vi "dospi_1394_grises.vi"() -> (0 "dt (ms) 2":u16=5, 1 "Canal 2":string="X", 2 "InterfaceName":string="cam0", 3 "Puerto 2":refnum<visa-resource-name>="COM2", 4 "Selección Rectángulo (px) 2":T1={"Left"=80, "Top"=180, "Right"=730, "Bottom"=830}, 5 "V 2Pi\nActual":sgl=3.4309938 format="%#.1g")   [LabVIEW 2020]
uses:
  <vilib>/Instr/_visa.llb/VISA Find Search Mode.ctl
  <vilib>/Instr/_visa.llb/VISA Configure Serial Port (Instr).vi
  <vilib>/vision/NI_Vision_Development_Module.lvlib
  <vilib>/gmath/NI_Gmath.lvlib
  <vilib>/vision/driver/NI_Vision_Acquisition_Software.lvlib
  <vilib>/Analysis/NI_AAL_SigProc.lvlib
panel:
  in  "Sust":bool=TRUE
  in  "Sustracción 2":bool
  in  "V 2Pi\nApriori":sgl=4.0 min=0.1 max=15 step=0.1 format="%.1f"
  in  "Puerto":refnum<visa-resource-name>="COM2"
  in  "Selección Rectángulo (px)":T1={"Left"=80, "Top"=180, "Right"=730, "Bottom"=830}
  in  "dV (V)":sgl=0.4 min=0.1 max=5 step=0.1 format="%.1f"
  in  "dt (ms)":u16=5
  in  "Rango (V)":u8=7 max=100 step=1
  in  "Canal":string="X"
  out "valor enviado":string="17.2"
  in  "Sustracción":bool
  out "Captura":T2(plugin-control)
  in  "error in (no error)":errorcluster
  out "tiempo total":u32=1016
  out "Ciclos 2Pi":cluster{"xi used":dbl[], "yi":dbl[]}[](graph)=[{"xi used"=[0.0, 0.4000000059604645, 0.800000011920929, 1.2000000476837158, 1.600000023841858, 2.0, 2.4000000953674316, 2.799999952316284, 3.200000047683716, 3.6000001430511475, 4.0, 4.400000095367432, 4.800000190734863, 5.200000286102295, 5.599999904632568, 6.0, 6.400000095367432, 6.800000190734863, 7.200000286102295], "yi"=[1.6194082498550415, 2.081223726272583, 3.9639101028442383, 5.417988300323486, 5.994996547698975, 5.763517379760742, 4.927460193634033, 3.268064022064209, 1.9228070974349976, 2.006049633026123, 3.322584629058838, 5.178757190704346, 5.874281883239746, 5.9817633628845215, 5.3586106300354, 3.7743194103240967, 2.4187028408050537, 2.3153183460235596, 3.7917206287384033]}, {"xi used"=[0.0, 0.10000000149011612, 0.20000000298023224, 0.30000000447034836, 0.4000000059604645, 0.5000000074505806, 0.6000000089406967, 0.7000000104308128, 0.800000011920929, 0.9000000208616257, 1.0000000298023224, 1.100000038743019, 1.2000000476837158, 1.3000000417232513, 1.4000000357627869, 1.5000000298023224, 1.600000023841858, 1.7000000178813934, 1.800000011920929, 1.9000000059604645, 2.0, 2.100000023841858, 2.200000047683716, 2.3000000715255737, 2.4000000953674316, 2.5000000596046448, 2.600000023841858, 2.699999988079071, 2.799999952316284, 2.899999976158142, 3.0, 3.100000023841858, 3.200000047683716, 3.3000000715255737, 3.4000000953674316, 3.5000001192092896, 3.6000001430511475, 3.7000001072883606, 3.8000000715255737, 3.900000035762787, 4.0, 4.100000023841858, 4.200000047683716, 4.300000071525574, 4.400000095367432, 4.5000001192092896, 4.6000001430511475, 4.700000166893005, 4.800000190734863, 4.900000214576721, 5.000000238418579, 5.100000262260437, 5.200000286102295, 5.300000190734863, 5.400000095367432, 5.5, 5.599999904632568, 5.699999928474426, 5.799999952316284, 5.899999976158142, 6.0, 6.100000023841858, 6.200000047683716, 6.300000071525574, 6.400000095367432, 6.5000001192092896, 6.6000001430511475, 6.700000166893005, 6.800000190734863, 6.900000214576721, 7.000000238418579, 7.100000262260437, 7.200000286102295], "yi"=[1.6194082498550415, 1.6415202646400873, 1.700969021152869, 1.835091261121122, 2.081223726272583, 2.4615675244221595, 2.9377812277334487, 3.4563877744572187, 3.9639101028442383, 4.416314498578613, 4.807340439884618, 5.1401707620402455, 5.417988300323486, 5.643229129866736, 5.815342479071086, 5.9330308007455095, 5.994996547698975, 6.0015645873541725, 5.959549445588673, 5.8773880628937665, 5.763517379760742, 5.622745854472534, 5.4453682711596425, 5.218050945615625, 4.927460193634033, 4.566549653810085, 4.153420905030226, 3.7124627576598135, 3.268064022064209, 2.8442846434260165, 2.4638706226251452, 2.1492390703865025, 1.9228070974349976, 1.8016579460584699, 1.7815393847964844, 1.8528653137515367, 2.006049633026123, 2.2327082258196134, 2.529265762805696, 2.8933489839101707, 3.322584629058838, 3.807336769827714, 4.308917005977046, 4.78137419407865, 5.178757190704346, 5.467236063197128, 5.661465721984701, 5.788222288265946, 5.874281883239746, 5.940712665430707, 5.985750942666336, 6.001925060099863, 5.9817633628845215, 5.9173299887642, 5.798831744986865, 5.616011126946077, 5.3586106300354, 5.0225638976458455, 4.628571701943094, 4.203526165358669, 3.7743194103240967, 3.3657338746848104, 2.994113257941885, 2.673691575010305, 2.4187028408050537, 2.2430304554985607, 2.1591553602930404, 2.1792078816481535, 2.3153183460235596, 2.5722541809073114, 2.925331217901028, 3.3425023896347215, 3.7917206287384033]}, {"xi used"=[1.6635191881348852, 5.094512955533968], "yi"=[6.004797437208987, 6.001979760925586]}]
  out "error out":errorcluster
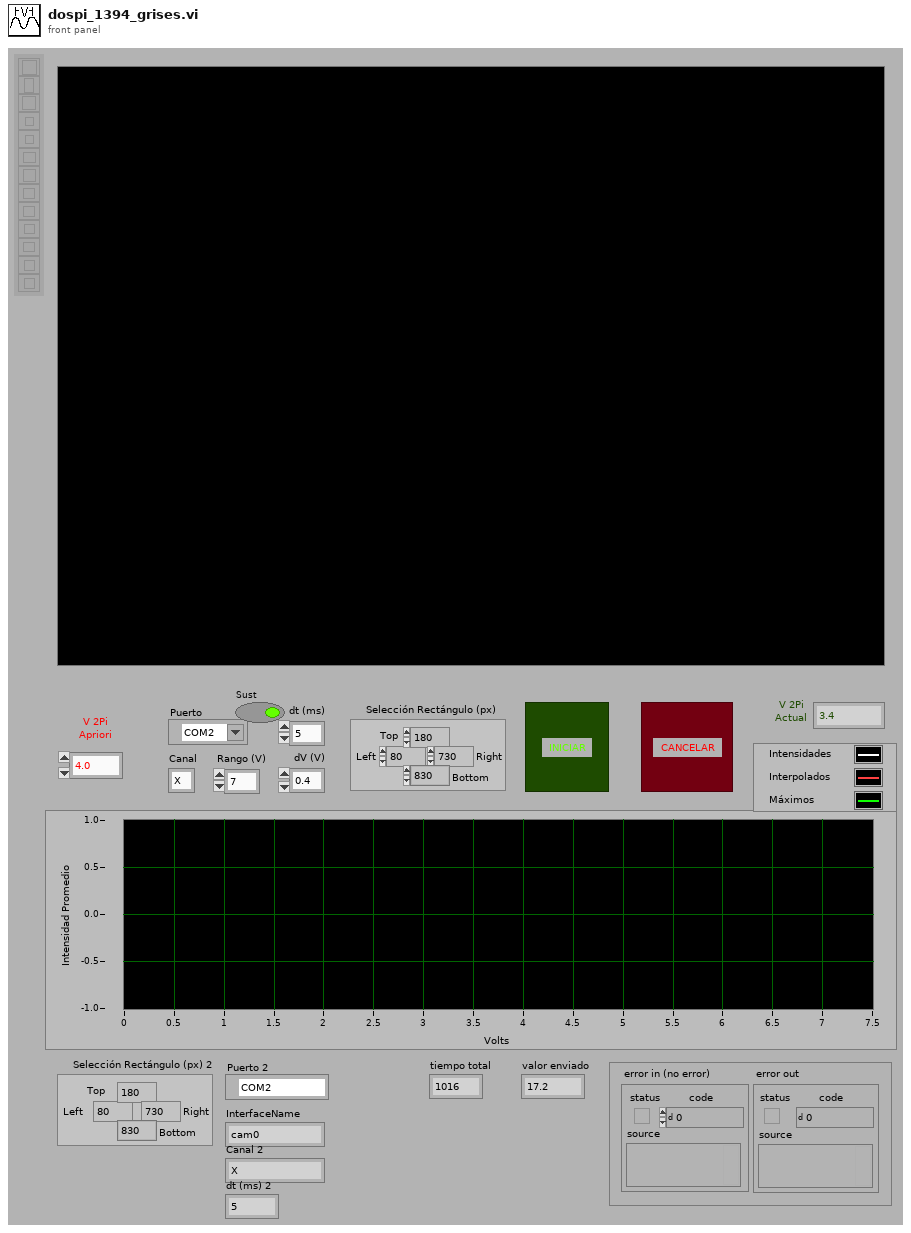
[diagram p1: front panel]
types:
  T1 = cluster{"Left":i32, "Top":i32, "Right":i32, "Bottom":i32}
  T2 = typedef "IMAQ Image.ctl" = refnum<image>
  T3 = typedef "VISA Find Search Mode.ctl" = u32
  T4 = cluster{"Type":u32, "Version":u32, "Flags":u32, "SerialNumberHigh":u32, "SerialNumberLow":u32, "BusType":u32, "InterfaceName":string, "VendorName":string, "ModelName":string, "CameraFileName":string, "CameraAttributeURL":string}[]
  T5 = cluster{"Type":u32, "Version":u32, "Flags":u32, "SerialNumberHigh":u32, "SerialNumberLow":u32, "BusType":u32, "InterfaceName":string, "VendorName":string, "ModelName":string, "CameraFileName":string, "CameraAttributeURL":string}
  T6 = typedef "IMAQdx.ctl" = refnum<k21>
  T7 = cluster{"Mean Value":sgl, "Standard Variation":sgl, "Minimal Value":sgl, "Maximal Value":sgl, "Area (calibrated)":sgl, "Area (pixels)":i32, "%":sgl}
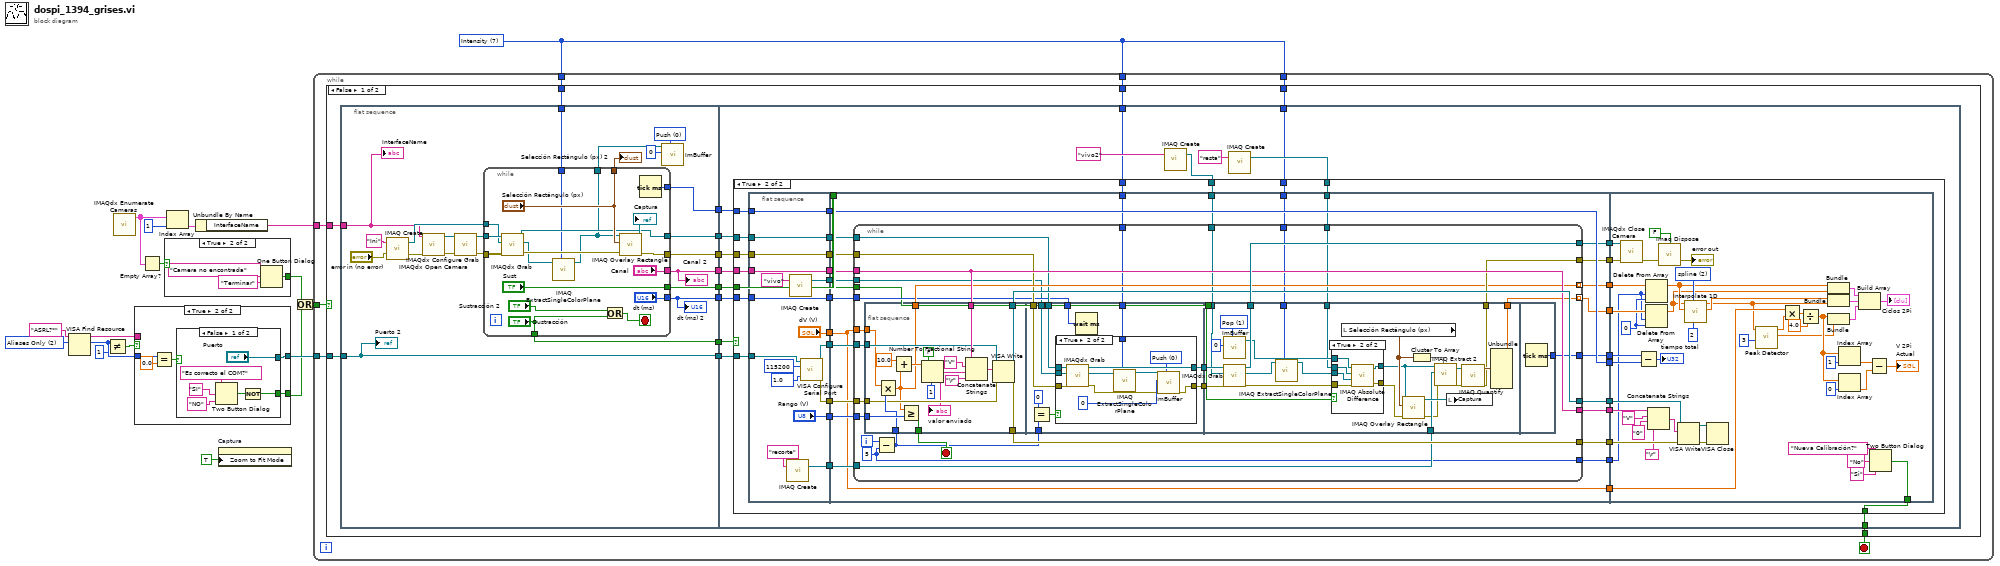
[diagram p0: block diagram]
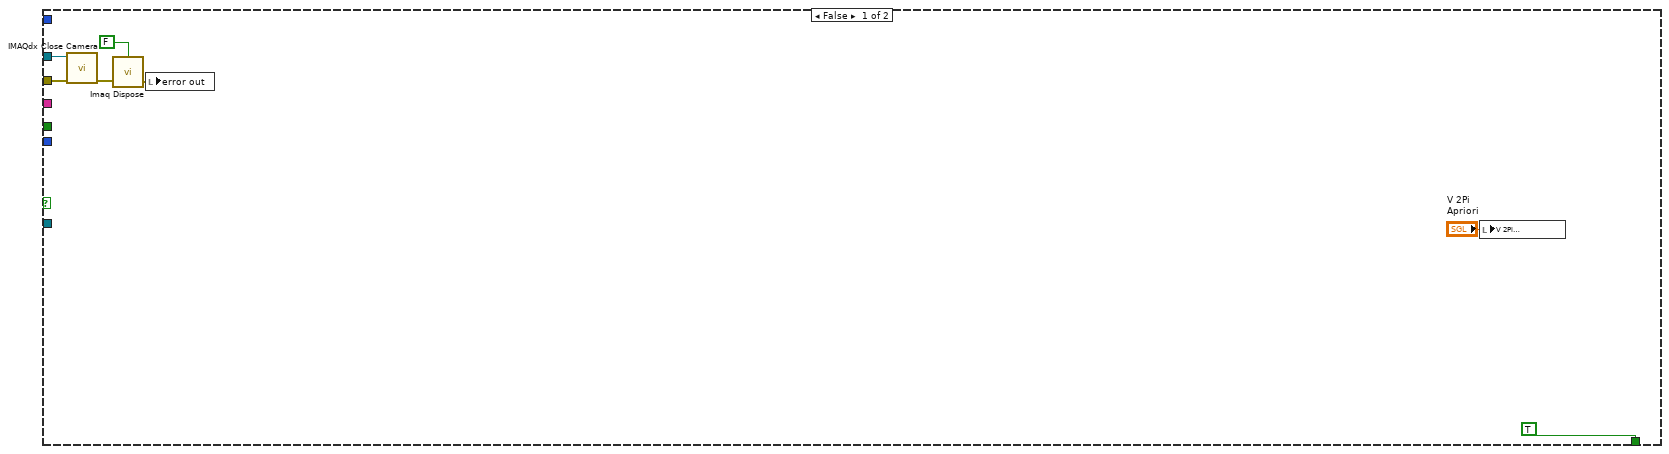
[diagram p2: hidden frame]
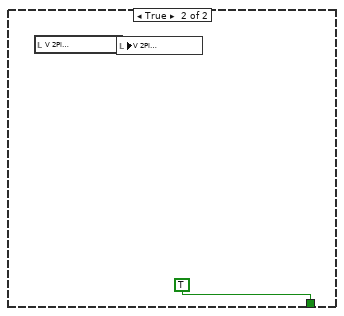
[diagram p5: hidden frame]
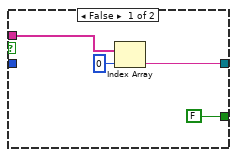
[diagram p6: hidden frame]
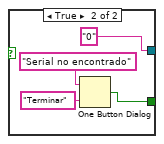
[diagram p7: hidden frame]
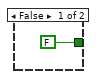
[diagram p8: hidden frame]
diagram:
  w1 = 7 items=["Red", "Green", "Blue", "Hue", "Saturation", "Luminance", "Value", "Intensity"] ("Color Plane")
  w12 = T3 2 items=["Canonical Names Only"=0, "Aliases Only"=2, "Include Matching Aliases"=3, "Include All Aliases"=4] ("Search Mode")
  n1 = VISA Find Resource(10:w12, 11:"ASRL?*" ("expression (\"?*\")")) -> (2:w17:u32, 3:w16:string[])  [unwired: 1 in, 1 out]
  n2 = Not Equal?(x=w17, y=u32 1) -> (x != y?=w15:bool)
  n3 = call <vilib>:"IMAQdx Enumerate Cameras.vi"() -> ("Camera Information Array"=w10:T4)  [unwired: 10 in, 1 out]
  n4 = case shown="True" w15 {
    tunnel: w16 -> [w21 _]
    tunnel: [w19 w26] -> w6
    tunnel: w17 -> [_ w24]
    tunnel: [FALSE ("true") w22] -> w4
    frame False {
      n5 = Index Array(array=w21, index=0) -> (element=w19:string)
    }
    frame True {
      n6 = Equal?(x=w24, y=0.0) -> (x = y?=w23:bool)
      n7 = case shown="False" w23 {
        tunnel: ["Puerto" "0" ("button name (\"OK\")")] -> w26
        tunnel: [w27 w33] -> w22
        frame False {
          n8 = Two Button Dialog(message="Es correcto el COM?" ("error source (\" \")"), 1:"NO" ("F button name (\"Cancel\")"), 2:"SI" ("T button name (\"OK\")")) -> (T button?=w28:bool)
          n9 = Not(x=w28) -> (.not. x?=w27:bool)
        }
        frame True {
          n10 = One Button Dialog(message="Serial no encontrado" ("error source (\" \")"), button name ("OK")="Terminar") -> (true=w33:bool)
        }
      }
    }
  }
  n11 = Empty Array?(array=w10) -> (empty?=w11:bool)
  n12 = case shown="True" w11 {
    tunnel: [FALSE ("true") w38] -> w5
    frame False {
    }
    frame True {
      n13 = One Button Dialog(message="Camera no encontrada" ("error source (\" \")"), button name ("OK")="Terminar") -> (true=w38:bool)
    }
  }
  n14 = Index Array(array=w10, index=1) -> (element=w9:T5)
  n15 = Unbundle By Name(w9) -> ("InterfaceName"=w7:string)
  n16 = property on="Captura" class="ImageControl"("Zoom to Fit Mode"=TRUE) -> ()  [unwired: 2 in, 2 out]
  n17 = Or(x=w5, y=w4) -> (x .or. y?=w3:bool)
  n18 = while {
    tunnel: w7 -> [w47]
    tunnel: w6 -> [w46]
    tunnel: w3 -> [w45]
    tunnel: w1 -> [w43]
    tunnel: w1 -> [w42]
    tunnel: w1 -> [w41]
    stop <- w44 stop-if-true
    n19 = case shown="False" w45 {
      tunnel: w47 -> [w61 _]
      tunnel: w46 -> [w60 _]
      tunnel: [w52 TRUE ("T button?")] -> w44
      tunnel: w43 -> [w50 _]
      tunnel: w42 -> [w49 _]
      tunnel: w41 -> [w48 _]
      frame False {
        n20 = flat-sequence {
          tunnel: w61 -> [w75]
          tunnel: w60 -> [w68]
          tunnel: [w68] -> w59
          tunnel: [w74] -> w58
          tunnel: [w73] -> w57
          tunnel: [w72] -> w56
          tunnel: [w71] -> w55
          tunnel: [w70] -> w54
          tunnel: [w69] -> w53
          tunnel: [w63] -> w51
          tunnel: w50 -> [w62]
          tunnel: w59 -> [w116]
          tunnel: w58 -> [w115]
          tunnel: w57 -> [w114]
          tunnel: w56 -> [w113]
          tunnel: w55 -> [w112]
          tunnel: w54 -> [w111]
          tunnel: w53 -> [w110]
          tunnel: [w109] -> w52
          tunnel: w51 -> [w104]
          tunnel: w49 -> [w103]
          tunnel: w48 -> [w102]
          frame #0 {
            w65 = u16 0 items=["Push", "Pop", "Reset"] ("Function")
            n21 = call "IMAQ Create"("Image Name"="Ini", "error in (no error)"="error in (no error)") -> ("New Image"=w79:T2, "error out"=w76:errorcluster)  [unwired: 3 in]
            n22 = call <vilib>:"IMAQdx Open Camera.vi"("error in"=w76, "Session In"=w75) -> ("error out"=w77:errorcluster, "Session Out"=w78:T6)  [unwired: 8 in]
            n23 = call <vilib>:"IMAQdx Configure Grab.vi"("error in"=w77, "Session In"=w78) -> ("error out"=w80:errorcluster, "Session Out"=w81:T6)  [unwired: 8 in]
            n24 = while {
              tunnel: w80 -> [w100]
              tunnel: [w89] -> w73
              tunnel: w81 -> [w101]
              tunnel: w79 -> [w99]
              tunnel: [w98] -> w74
              tunnel: [w91] -> w72
              tunnel: ["Sustracción"] -> w71
              tunnel: ["Canal"] -> w70
              tunnel: ["dt (ms)"] -> w69
              tunnel: [w85] -> w66
              tunnel: ["Selección Rectángulo (px)"] -> w67
              tunnel: ["Sust"] -> w63
              tunnel: w62 -> [w84]
              stop <- w97 stop-if-true
              n25 = call <vilib>:"IMAQdx Grab.vi"("error in"=w100, "Image In"=w99, "Session In"=w101) -> ("error out"=w87:errorcluster, "Image Out"=w86:T2, "Session Out"=w89:T6)  [unwired: 5 in, 1 out]
              n26 = call "IMAQ ExtractSingleColorPlane"("Color Plane"=w84, "Image Src"=w86) -> ("Image Dst Out"=w85:T2)  [unwired: 8 in, 1 out]
              n27 = Or(x="Sustracción 2", y="Sustracción") -> (x .or. y?=w97:bool)
              n28 = call "IMAQ Overlay Rectangle"("error in (no error)"=w87, "Rectangle"="Selección Rectángulo (px)", "Image"=w85) -> ("error out"=w91:errorcluster, "Image Out"=→"Captura":T2)  [unwired: 7 in]
              n29 = Tick Count (ms)() -> (millisecond timer value=w98:u32)
            }
            "Canal 2" <- w70
            "dt (ms) 2" <- w69
            "Selección Rectángulo (px) 2" <- w67
            n30 = call "ImBuffer.vi"("Function"=w65, "Buffer #"=0, "Image In"=w66) -> ()  [unwired: 6 in, 3 out]
            "Puerto 2" <- w68
            "InterfaceName" <- w75
          }
          frame #1 {
            n31 = call "IMAQ Create"("Image Name"="vivo2") -> ("New Image"=w105:T2)  [unwired: 4 in, 1 out]
            n32 = call "IMAQ Create"("Image Name"="resta") -> ("New Image"=w107:T2)  [unwired: 4 in, 1 out]
            n33 = case shown="True" w112 {
              tunnel: w116 -> [_ w136]
              tunnel: w115 -> [_ w135]
              tunnel: w114 -> [w123 w134]
              tunnel: w113 -> [w122 w133]
              tunnel: w111 -> [_ w132]
              tunnel: w110 -> [_ w130]
              tunnel: [TRUE ("T button?") w129] -> w109
              tunnel: w107 -> [_ w128]
              tunnel: w105 -> [_ w127]
              tunnel: w104 -> [_ w126]
              tunnel: w103 -> [_ w125]
              tunnel: w102 -> [_ w124]
              frame False {
                n34 = call <vilib>:"IMAQdx Close Camera.vi"("error in"=w122, "Session In"=w123) -> ("error out"=w119:errorcluster)  [unwired: 9 in]
                n35 = call "Imaq Dispose"("All Images? (No)"=FALSE, "error in (no error)"=w119) -> ("error out"=w117:errorcluster)  [unwired: 4 in]
                n36 = local write "error out"(w117) -> ()
                n37 = local write "V 2Pi\nActual"("V 2Pi\nApriori") -> ()
              }
              frame True {
                n38 = flat-sequence {
                  tunnel: ["Rango (V)"] -> w157
                  tunnel: [w158] -> w156
                  tunnel: [w163] -> w155
                  tunnel: [w162] -> w154
                  tunnel: [w164] -> w153
                  tunnel: [w166] -> w152
                  tunnel: [w161] -> w151
                  tunnel: [w169] -> w150
                  tunnel: [w168] -> w149
                  tunnel: ["dV (V)"] -> w148
                  tunnel: w136 -> [w165]
                  tunnel: w135 -> [w164]
                  tunnel: w134 -> [w163]
                  tunnel: w133 -> [w162]
                  tunnel: w132 -> [w161]
                  tunnel: [w160] -> w131
                  tunnel: w130 -> [w160]
                  tunnel: w157 -> [w181]
                  tunnel: w156 -> [w197]
                  tunnel: w155 -> [w198]
                  tunnel: w154 -> [w196]
                  tunnel: w153 -> [w195]
                  tunnel: [w195] -> w147
                  tunnel: [w194] -> w146
                  tunnel: [w193] -> w145
                  tunnel: [w192] -> w144
                  tunnel: [w191] -> w143
                  tunnel: [w190] -> w142
                  tunnel: [w189] -> w141
                  tunnel: [w188] -> w140
                  tunnel: [w187] -> w139
                  tunnel: w152 -> [w186]
                  tunnel: w151 -> [w185]
                  tunnel: w150 -> [w183]
                  tunnel: w149 -> [w184]
                  tunnel: [w182] -> w138
                  tunnel: w148 -> [w180]
                  tunnel: [w180] -> w137
                  tunnel: w131 -> [w179]
                  tunnel: w128 -> [w178]
                  tunnel: w127 -> [w177]
                  tunnel: w126 -> [w176]
                  tunnel: w125 -> [w175]
                  tunnel: w124 -> [w174]
                  tunnel: w147 -> [w343]
                  tunnel: w146 -> [w347]
                  tunnel: w145 -> [w346]
                  tunnel: w144 -> [w345]
                  tunnel: w143 -> [w344]
                  tunnel: w142 -> [w333]
                  tunnel: w141 -> [w341]
                  tunnel: w140 -> [w342]
                  tunnel: w139 -> [w335]
                  tunnel: w138 -> [w331]
                  tunnel: w137 -> [w328]
                  tunnel: [w313] -> w129
                  frame #0 {
                    w171 = u16 10 items=["1.0"=10, "1.5"=15, "2.0"=20] ("stop bits (10: 1 bit)")
                    n39 = call "IMAQ Create"("Image Name"="recorte") -> ("New Image"=w166:T2)  [unwired: 4 in, 1 out]
                    n40 = call "IMAQ Create"("Image Name"="vivo") -> ("New Image"=w158:T2)  [unwired: 4 in, 1 out]
                    n41 = call-poly "VISA Configure Serial Port"("VISA resource name"=w165, "baud rate (9600)"=u32 115200, "stop bits (10: 1 bit)"=w171) -> ("VISA resource name out"=w168:refnum<visa-resource-name>, "error out"=w169:errorcluster)  [unwired: 11 in]
                  }
                  frame #1 {
                    n42 = while {
                      tunnel: [w217] -> w190 mode=indexing
                      tunnel: [w221] -> w194
                      tunnel: w185 -> [w221]
                      tunnel: [w222] -> w193
                      tunnel: w184 -> [w223]
                      tunnel: w183 -> [w224]
                      tunnel: w181 -> [w225]
                      tunnel: [w226] -> w192
                      tunnel: w196 -> [w207]
                      tunnel: w197 -> [w203]
                      tunnel: w198 -> [w208]
                      tunnel: [w220] -> w191
                      tunnel: [w214] -> w189
                      tunnel: [w219] -> w188
                      tunnel: [w218] -> w187 mode=indexing
                      tunnel: w186 -> [w216]
                      tunnel: [w212] -> w182
                      tunnel: w180 -> [w211]
                      tunnel: w179 -> [w204]
                      tunnel: w178 -> [w210]
                      tunnel: w177 -> [w202]
                      tunnel: w176 -> [w201]
                      tunnel: w175 -> [w200]
                      tunnel: w174 -> [w199]
                      i -> [w213]
                      stop <- w215 stop-if-true
                      w212 = 5 ("x")
                      n43 = flat-sequence {
                        tunnel: w223 -> [w231]
                        tunnel: w224 -> [w234]
                        tunnel: [w242] -> w215
                        tunnel: w209 -> [w239]
                        tunnel: w225 -> [w241]
                        tunnel: w221 -> [w233]
                        tunnel: [w227] -> w218
                        tunnel: [w230] -> w222
                        tunnel: [w229] -> w219
                        tunnel: w211 -> [w228]
                        tunnel: w204 -> [w254]
                        tunnel: w209 -> [w252]
                        tunnel: w208 -> [w250]
                        tunnel: w207 -> [w249]
                        tunnel: [w248] -> w206
                        tunnel: [w247] -> w205
                        tunnel: w203 -> [w246]
                        tunnel: w200 -> [w245]
                        tunnel: [w288] -> w226
                        tunnel: [w287] -> w220
                        tunnel: [w286] -> w217
                        tunnel: w216 -> [w285]
                        tunnel: w210 -> [w275]
                        tunnel: w206 -> [w281]
                        tunnel: w205 -> [w280]
                        tunnel: w202 -> [w277]
                        tunnel: w201 -> [w272]
                        tunnel: w199 -> [w268]
                        tunnel: [w301] -> w214
                        frame #0 {
                          n44 = Multiply(x=w228, y=w239) -> (x*y=w227:sgl)
                          n45 = Add(x=sgl 10.0, y=w227) -> (x+y=w244:sgl)
                          n46 = Greater Or Equal?(x=w227, y=w241) -> (x >= y?=w242:bool)
                          n47 = Number To Fractional String(use system decimal point (T)=FALSE, number=w244, precision (6)=i16 1) -> (F-format string=w232:string)  [unwired: 1 in]
                          "valor enviado" <- w232
                          n48 = Concatenate Strings(w233, "V" ("Substring"), w232, "\r") -> (w237:string)
                          n49 = VISA Write(VISA resource name=w231, write buffer=w237, error in (no error)=w234) -> (VISA resource name out=w230:refnum<visa-resource-name>, error out=w229:errorcluster)  [unwired: 1 out]
                        }
                        frame #1 {
                          n50 = Equal?(x=u8 0 ("y"), y=w252) -> (x = y?=w253:bool)
                          n51 = case shown="True" w253 {
                            tunnel: w250 -> [w256 w267]
                            tunnel: [w256 w266] -> w247
                            tunnel: w249 -> [w255 w265]
                            tunnel: [w255 w263] -> w248
                            tunnel: w246 -> [_ w261]
                            tunnel: w245 -> [_ w257]
                            frame False {
                            }
                            frame True {
                              w262 = u16 0 items=["Push", "Pop", "Reset"] ("Function")
                              n52 = call <vilib>:"IMAQdx Grab.vi"("error in"=w265, "Image In"=w261, "Session In"=w267) -> ("error out"=w260:errorcluster, "Image Out"=w259:T2, "Session Out"=w266:T6)  [unwired: 5 in, 1 out]
                              n53 = call "IMAQ ExtractSingleColorPlane"("Color Plane"=w257, "Image Src"=w259) -> ("Image Dst Out"=w258:T2)  [unwired: 8 in, 1 out]
                              n54 = call "ImBuffer.vi"("Function"=w262, "error in (no error)"=w260, "Buffer #"=0, "Image In"=w258) -> ("error out"=w263:errorcluster)  [unwired: 5 in, 2 out]
                            }
                          }
                          n55 = Wait (ms)(milliseconds to wait=w254) -> ()  [unwired: 1 out]
                        }
                        frame #2 {
                          w278 = u16 1 items=["Push", "Pop", "Reset"] ("Function")
                          n56 = call "ImBuffer.vi"("Function"=w278, "Buffer #"=0) -> ("Image Out"=w276:T2)  [unwired: 7 in, 2 out]
                          n57 = call <vilib>:"IMAQdx Grab.vi"("error in"=w281, "Image In"=w277, "Session In"=w280) -> ("error out"=w271:errorcluster, "Image Out"=w270:T2, "Session Out"=w288:T6)  [unwired: 5 in, 1 out]
                          n58 = call "IMAQ ExtractSingleColorPlane"("Color Plane"=w268, "Image Src"=w270) -> ("Image Dst Out"=w269:T2)  [unwired: 8 in, 1 out]
                          n59 = case shown="True" w272 {
                            tunnel: w271 -> [w294 w300]
                            tunnel: w276 -> [_ w299]
                            tunnel: w269 -> [w293 w298]
                            tunnel: w275 -> [_ w297]
                            tunnel: [w294 w296] -> w274
                            tunnel: [w293 w295] -> w273
                            frame False {
                            }
                            frame True {
                              n60 = call "IMAQ Absolute Difference"("Image Src A"=w299, "Image Dst"=w297, "Image Src B"=w298, "error in (no error)"=w300) -> ("Image Dst Out"=w295:T2, "error out"=w296:errorcluster)  [unwired: 3 in]
                            }
                          }
                          n61 = local read "Selección Rectángulo (px)"() -> (w289:T1)
                          n62 = call "IMAQ Overlay Rectangle"("error in (no error)"=w274, "Rectangle"=w289, "Image"=w273) -> ("error out"=w282:errorcluster, "Image Out"=w290:T2)  [unwired: 7 in]
                          n63 = Cluster To Array(cluster=w289) -> (array=w291:i32[])
                          n64 = call "IMAQ Extract 2"("Optional Rectangle"=w291, "error in (no error)"=w282, "Image Dst"=w285, "Image Src"=w273) -> ("error out"=w284:errorcluster, "Image Dst Out"=w283:T2)  [unwired: 6 in]
                          n65 = local write "Captura"(w290) -> ()
                          n66 = call "IMAQ Quantify"("error in (no error)"=w284, "Image"=w283) -> ("error out"=w287:errorcluster, "Global Report"=w292:T7)  [unwired: 1 in, 1 out]
                          n67 = Unbundle(w292) -> ("Mean Value"=w286:sgl)  [unwired: 6 out]
                        }
                        frame #3 {
                          n68 = Tick Count (ms)() -> (millisecond timer value=w301:u32)
                        }
                      }
                      n69 = Subtract(x=w213, y=w212) -> (x-y=w209:i32)
                    }
                  }
                  frame #2 {
                    w332 = 0 ("index")
                    w336 = 2 items=["nearest", "linear", "spline", "cubic Hermite", "Lagrange"] ("method")
                    n70 = call <vilib>:"IMAQdx Close Camera.vi"("error in"=w344, "Session In"=w345) -> ("error out"=w302:errorcluster)  [unwired: 9 in]
                    n71 = Subtract(x=w341, y=w343) -> (x-y=→"tiempo total":u32)
                    n72 = Delete From Array(array=w335, length=w331, index=w332) -> (array with subset deleted=w334:sgl[])  [unwired: 1 out]
                    n73 = Delete From Array(array=w333, length=w331, index=w332) -> (array with subset deleted=w330:sgl[])  [unwired: 1 out]
                    n74 = Concatenate Strings(w347, "V" ("Substring"), "0" ("Substring"), "\r") -> (w324:string)
                    n75 = call "Imaq Dispose"("All Images? (No)"=FALSE, "error in (no error)"=w302) -> ("error out"=→"error out":errorcluster)  [unwired: 4 in]
                    n76 = VISA Write(VISA resource name=w346, write buffer=w324, error in (no error)=w342) -> (VISA resource name out=w322:refnum<visa-resource-name>, error out=w323:errorcluster)  [unwired: 1 out]
                    n77 = call <vilib>:"Interpolate 1D.vi"("ntimes"=2, "method"=w336, "X"=w334, "Y"=w330) -> ("xi used"=w321:dbl[], "yi"=w308:dbl[])  [unwired: 5 in, 1 out]
                    n78 = VISA Close(VISA resource name=w322, error in (no error)=w323) -> ()  [unwired: 1 out]
                    n79 = call <vilib>:"Peak Detector.vi"("width"=3, "X"=w308) -> ("Amplitudes"=w306:dbl[], "Locations"=w307:dbl[])  [unwired: 5 in, 3 out]
                    n80 = Multiply(x=w328, y=w307) -> (x*y=w320:dbl[])
                    n81 = Divide(x=w320, y=sgl 4.0 ("x")) -> (x/y=w316:dbl[])
                    n82 = Bundle(w334, w330) -> (w339:cluster{sgl[], sgl[]})  [unwired: 1 in]
                    n83 = Bundle("xi used"=w321, "yi"=w308) -> (w338:cluster{"xi used":dbl[], "yi":dbl[]})  [unwired: 1 in]
                    n84 = Bundle(w316, "Amplitudes"=w306) -> (w329:cluster{dbl[], "Amplitudes":dbl[]})  [unwired: 1 in]
                    n85 = Index Array(array=w316, index=1) -> (element=w315:dbl)
                    n86 = Index Array(array=w316, index=0) -> (element=w314:dbl)
                    n87 = Build Array(w339, w338, w329) -> (→"Ciclos 2Pi":cluster{"xi used":dbl[], "Amplitudes":dbl[]}[])
                    n88 = Subtract(x=w315, y=w314) -> (x-y=→"V 2Pi\nActual":dbl)
                    n89 = Two Button Dialog(message="Nueva Calibración?", 1:"Si" ("F button name (\"Cancel\")"), 2:"No" ("F button name (\"Cancel\")")) -> (T button?=w313:bool)
                  }
                }
              }
            }
          }
        }
      }
      frame True {
        n90 = local read "V 2Pi\nApriori"() -> (w349:sgl)
        n91 = local write "V 2Pi\nActual"(w349) -> ()
      }
    }
  }
